vi "Read TEDS Memory.vi"(11 "ILC in":refnum<class "ILC.lvclass">) -> (2 "TEDS Memory":T1, 3 "ILC out":refnum<class "ILC.lvclass">)   [LabVIEW 2015, in "ILCCommon.lvlib" / "ILC.lvclass"]
uses:
  <userlib>/Common/ILC/ILC/ILC.lvclass
  <userlib>/Common/ILC/Typedefs/TEDSMemory.ctl
  <userlib>/Common/ILC/ILC/ILC.lvclass/ILC.ctl
  <userlib>/Common/ILC/Typedefs/ILCTypedefs.lvlib
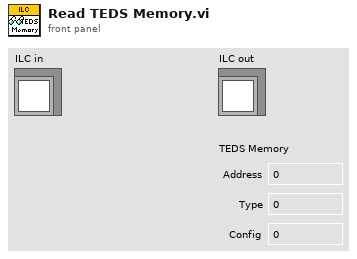
[diagram p1: front panel]
types:
  T1 = typedef "ILCCommon.lvlib/ILCTypedefs.lvlib/TEDSMemory.ctl" = cluster{"Address":i32, "Type":i32, "Config":i32}
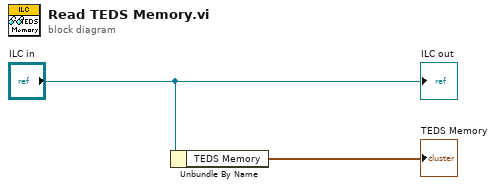
[diagram p0: block diagram]
diagram:
  n1 = Unbundle By Name("ILC in") -> ("TEDS Memory"=→"TEDS Memory":T1)
  "ILC out" <- "ILC in"
